vi "Autonomous Independent.vi"() -> ()   [LabVIEW 2017]
doc: "This VI is called when autonomous begins, and will automatically be terminated when autonomous ends. You can carry out timed or sensor driven robot movement independently without needing to return to the caller."
uses:
  <vilib>/Rock Robotics/WPI/RobotDrive/WPI_RobotDriveArcadeDrive_Standard(NoSaturation).vi
  <vilib>/Rock Robotics/Network Tables/NT Read String.vi
  <vilib>/Rock Robotics/Network Tables/NT Write Numeric Array.vi
  <vilib>/Rock Robotics/WPI/ThirdParty/Phoenix-LabVIEW/Motor Controller/Controls/CTRE_Phoenix_MotorControl_FeedbackDevice.ctl
  <vilib>/Rock Robotics/WPI/ThirdParty/Phoenix-LabVIEW/Motor Controller/Controls/CTRE_Phoenix_MotorControl_ControlMode.ctl
panel:
  in  "Output":dbl
  in  "milliseconds to wait":u32
  in  "Acceleration 2":i32
  in  "Cruise Velocity 2":i32
  in  "Invert? Right":bool
  in  "Invert? Left":bool
  in  "Right SensorPhase":bool
  in  "Left SensorPhase":bool
  in  "PIDF":cluster{"P":dbl, "I":dbl, "D":dbl, "F":dbl}
  # "Be sure to right-click and choose Data Operations>>Make Current Value default if you want to save the array values with the VI"
  # "Move 1"
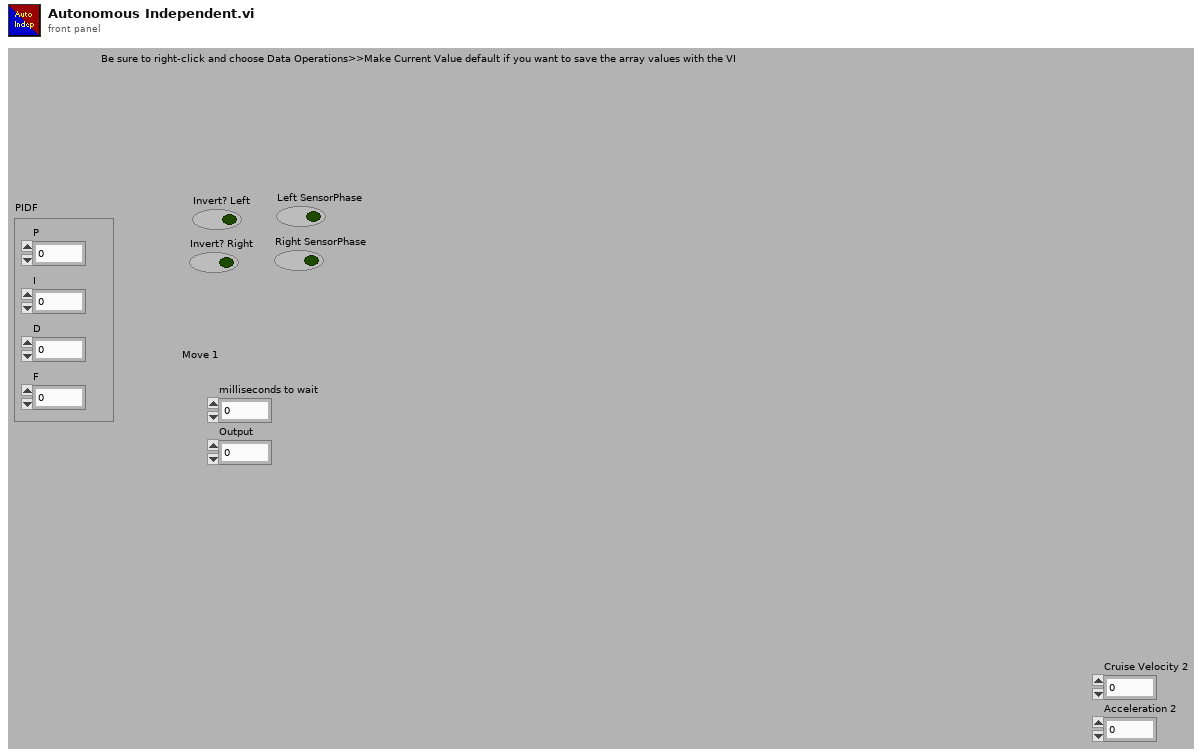
[diagram p1: front panel]
types:
  T1 = typedef "WPI_JoystickDevRef.ctl" = cluster{"Device":T2}
  T2 = typedef "WPI_JoystickDeviceEnum.ctl" = enum16{"USB 0", "USB 1", "USB 2", "USB 3", "USB 4", "USB 5"}
  T3 = typedef "WPI_MotorControlDeviceRef.ctl" = cluster{"DeviceStatus":errorcluster, "Type":T4, "PWM":cluster{"PWM Channel":T5, "DeadBand":T6}, "CAN":cluster{"Device Number":u8, "SetOutput VI Ref":variant, "GetOutput VI Ref":variant, "Enable VI Ref":variant, "Disable VI Ref":variant, "Data":variant}, "Invert":bool, "DIO PWM":cluster{"PWM \"Enable\" Channel":T5, "DIOChannel":T7, "PWM Rate":dbl}}
  T4 = typedef "WPI_MotorControlType.ctl" = enum16{"PWM", "CAN", "DIO PWM"}
  T5 = typedef "FPGA_DIOPWMChannel.ctl" = enum8{"PWM 0", "PWM 1", "PWM 2", "PWM 3", "PWM 4", "PWM 5", "PWM 6", "PWM 7", "PWM 8", "PWM 9", "PWM MXP 0", "PWM MXP 1", "PWM MXP 2", "PWM MXP 3", "PWM MXP 4", "PWM MXP 5", "PWM MXP 6", "PWM MXP 7", "PWM MXP 8", "PWM MXP 9", "Invalid"}
  T6 = typedef "WPI_PWMDeadband.ctl" = cluster{"Name":string, "maxPositivePwm":i32, "minPositivePwm":i32, "centerPwm":i32, "maxNegativePwm":i32, "minNegativePwm":i32, "angularRange":u16}
  T7 = typedef "FPGA_DIOChannel.ctl" = enum8{"DIO 0", "DIO 1", "DIO 2", "DIO 3", "DIO 4", "DIO 5", "DIO 6", "DIO 7", "DIO 8", "DIO 9", "DIO MXP 0", "DIO MXP 1", "DIO MXP 2", "DIO MXP 3", "DIO MXP 4", "DIO MXP 5", "DIO MXP 6", "DIO MXP 7", "DIO MXP 8", "DIO MXP 9", "DIO MXP 10", "DIO MXP 11", "DIO MXP 12", "DIO MXP 13", "DIO MXP 14", "DIO MXP 15", "SPI Port CS1", "SPI Port CS2", "SPI Port CS3", "SPI Port MISO", "SPI Port MOSI", "Invalid"}
  T8 = typedef "CTRE_Phoenix_MotorControl_FeedbackDevice.ctl" = i8
  T9 = typedef "CTRE_Phoenix_MotorControl_ControlMode.ctl" = u16
  T10 = typedef "WPI_RobotDriveDevRef.ctl" = cluster{"DevStatus":errorcluster, "Motors[]":T3[], "Square Inputs":bool, "Max Output":dbl}
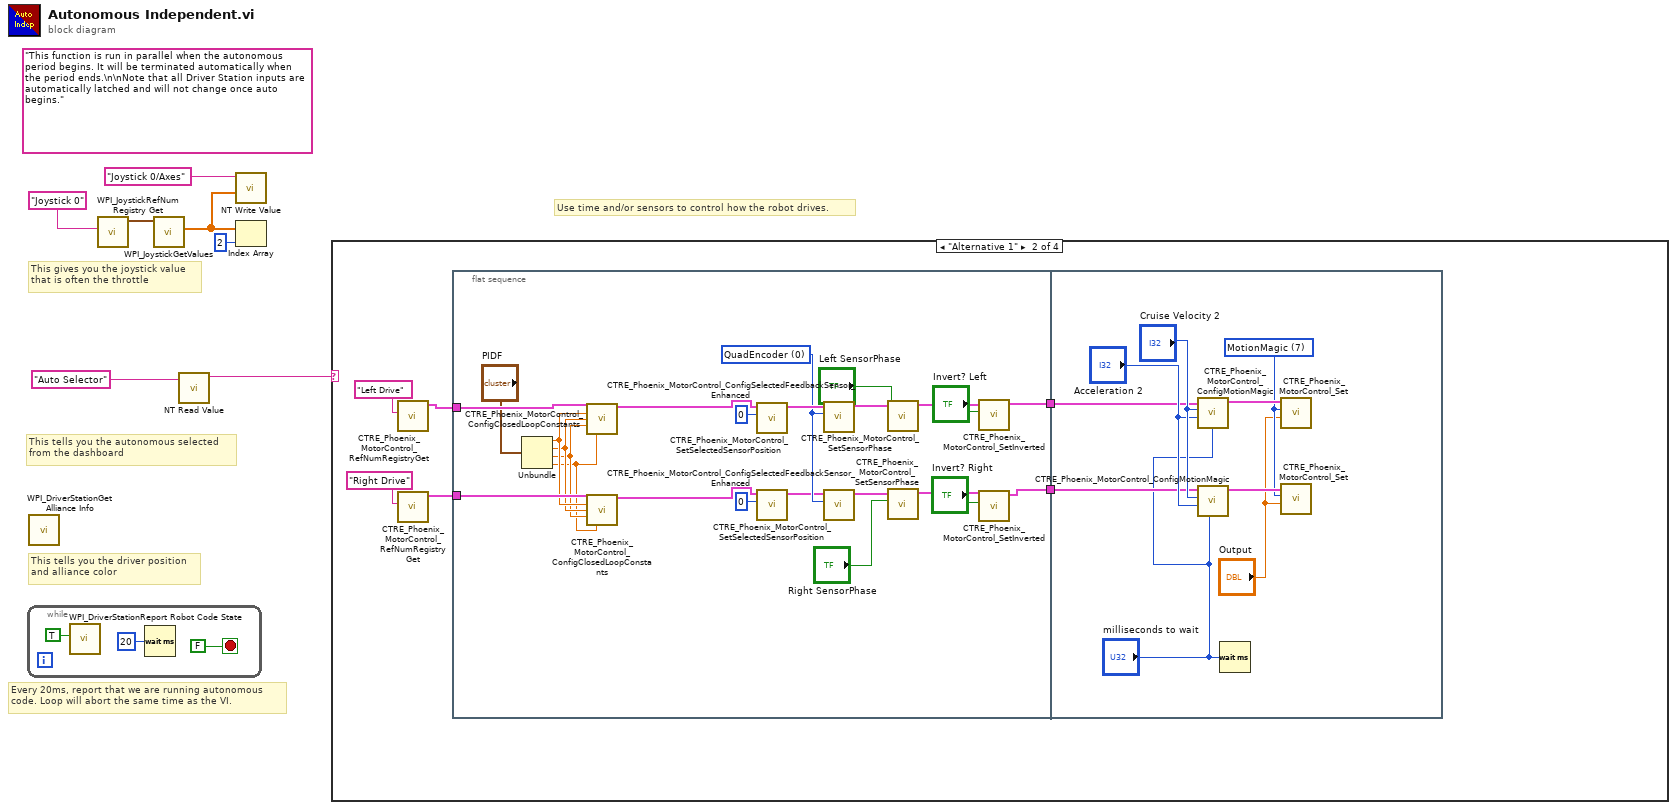
[diagram p0: block diagram]
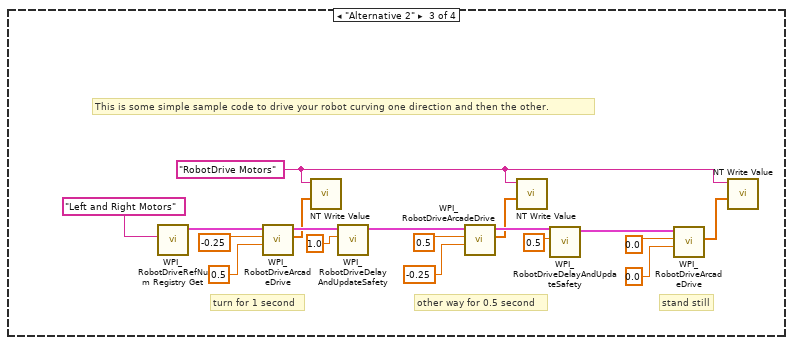
[diagram p3: hidden frame]
diagram:
  (unwired) "This function is run in parallel when the autonomous period begins. It will be terminated automatically when the period ends.\n\nNote that all Driver Station inputs are automatically latched and will not change once auto begins."
  # "This tells you the autonomous selected\nfrom the dashboard"
  # "Every 20ms, report that we are running autonomous\ncode. Loop will abort the same time as the VI."
  # "This gives you the joystick value\nthat is often the throttle"
  # "Use time and/or sensors to control how the robot drives."
  # "This tells you the driver position\nand alliance color"
  n1 = while {
    stop <- FALSE stop-if-true
    n2 = call <vilib>:"WPI_DriverStationReport Robot Code State.vi"("Autonomous"=TRUE) -> ()  [unwired: 10 in, 1 out]
    n3 = Wait (ms)(milliseconds to wait=u32 20) -> ()  [unwired: 1 out]
  }
  n4 = call <vilib>:"WPI_DriverStationGet Alliance Info.vi"() -> ()  [unwired: 12 out]
  n5 = call <vilib>:"WPI_JoystickRefNum Registry Get.vi"("refnum name"="Joystick 0") -> ("JoystickDevRef"=w6:T1)  [unwired: 1 in, 9 out]
  n6 = call <vilib>:"WPI_JoystickGetValues.vi"("JoystickDevRef"=w6) -> ("Axes"=w2:dbl[])  [unwired: 6 in, 4 out]
  n7 = call-poly <vilib>:"NT Read Value.vi"("Name"="Auto Selector") -> ("String"=w3:string)  [unwired: 9 in, 1 out]
  n8 = call-poly <vilib>:"NT Write Value.vi"("Numeric Array"=w2, "Name"="Joystick 0/Axes") -> ()  [unwired: 9 in, 1 out]
  n9 = Index Array(array=w2, index=2) -> ()  [unwired: 1 out]
  n10 = case shown="\"Alternative 1\"" w3 {
    frame Default {
      # "You can put your main auto here, or you can right-click on the case and make any\nother frame be the default case."
      # "This is the frame that will execute if no selection is made, or if it is not recognized"
    }
    frame "Alternative 1" {
      n11 = call <vilib>:"CTRE_Phoenix_MotorControl_RefNumRegistryGet.vi"("refnum name"="Left Drive") -> ("PhoenixMotorControlDevRef"=w14:T3)  [unwired: 9 in, 1 out]
      n12 = call <vilib>:"CTRE_Phoenix_MotorControl_RefNumRegistryGet.vi"("refnum name"="Right Drive") -> ("PhoenixMotorControlDevRef"=w13:T3)  [unwired: 9 in, 1 out]
      n13 = flat-sequence {
        tunnel: w14 -> [w40]
        tunnel: w13 -> [w39]
        tunnel: [w18] -> w12
        tunnel: [w17] -> w11
        tunnel: w12 -> [w47]
        tunnel: w11 -> [w46]
        frame #0 {
          w28 = T8 0 items=["None"=-1, "QuadEncoder"=0, "Analog"=2, "Tachometer"=4, "Pulse Width Encoded Position"=8, "Sensor Sum (S0 + S1)"=9, "Sensor Difference (D0 - D1)"=10, "Remote Source 0"=11, "Remote Source 1"=12, "Software Emulated"=15] ("Feedback Device")
          n14 = Unbundle("PIDF") -> ("P"=w37:dbl, "I"=w36:dbl, "D"=w35:dbl, "F"=w34:dbl)
          n15 = call <vilib>:"CTRE_Phoenix_MotorControl_ConfigClosedLoopConstants.vi"("PhoenixMotorControlDevRef"=w40, "P"=w37, "I"=w36, "D"=w35, "F"=w34) -> ("PhoenixMotorControlDevRef"=w33:T3)  [unwired: 9 in, 1 out]
          n16 = call <vilib>:"CTRE_Phoenix_MotorControl_ConfigClosedLoopConstants.vi"("PhoenixMotorControlDevRef"=w39, "P"=w37, "I"=w36, "D"=w35, "F"=w34) -> ("PhoenixMotorControlDevRef"=w32:T3)  [unwired: 9 in, 1 out]
          n17 = call "CTRE_Phoenix_MotorControl_SetSelectedSensorPosition.vi"("New Sensor Position"=0, "PhoenixMotorControlDevRef"=w33) -> ("PhoenixMotorControlDevRef"=w29:T3)  [unwired: 8 in, 1 out]
          n18 = call "CTRE_Phoenix_MotorControl_SetSelectedSensorPosition.vi"("New Sensor Position"=0, "PhoenixMotorControlDevRef"=w32) -> ("PhoenixMotorControlDevRef"=w27:T3)  [unwired: 8 in, 1 out]
          n19 = call <vilib>:"CTRE_Phoenix_MotorControl_ConfigSelectedFeedbackSensor_Enhanced.vi"("Feedback Device"=w28, "PhoenixMotorControlDevRef"=w29) -> ("PhoenixMotorControlDevRef"=w26:T3)  [unwired: 8 in, 1 out]
          n20 = call <vilib>:"CTRE_Phoenix_MotorControl_ConfigSelectedFeedbackSensor_Enhanced.vi"("Feedback Device"=w28, "PhoenixMotorControlDevRef"=w27) -> ("PhoenixMotorControlDevRef"=w25:T3)  [unwired: 8 in, 1 out]
          n21 = call <vilib>:"CTRE_Phoenix_MotorControl_SetSensorPhase.vi"("PhaseSensor"="Left SensorPhase", "PhoenixMotorControlDevRef"=w26) -> ("PhoenixMotorControlDevRef"=w21:T3)  [unwired: 8 in, 1 out]
          n22 = call <vilib>:"CTRE_Phoenix_MotorControl_SetSensorPhase.vi"("PhaseSensor"="Right SensorPhase", "PhoenixMotorControlDevRef"=w25) -> ("PhoenixMotorControlDevRef"=w22:T3)  [unwired: 8 in, 1 out]
          n23 = call <vilib>:"CTRE_Phoenix_MotorControl_SetInverted.vi"("Invert?"="Invert? Left", "PhoenixMotorControlDevRef"=w21) -> ("PhoenixMotorControlDevRef"=w18:T3)  [unwired: 8 in, 1 out]
          n24 = call <vilib>:"CTRE_Phoenix_MotorControl_SetInverted.vi"("Invert?"="Invert? Right", "PhoenixMotorControlDevRef"=w22) -> ("PhoenixMotorControlDevRef"=w17:T3)  [unwired: 8 in, 1 out]
        }
        frame #1 {
          w42 = T9 7 items=["PercentOutput"=0, "Position"=1, "Velocity"=2, "Current"=3, "Follower"=5, "MotionProfile"=6, "MotionMagic"=7, "MotionMagicArc"=8, "MotionProfileArc"=10, "Disabled"=15] ("Control Mode")
          n25 = call <vilib>:"CTRE_Phoenix_MotorControl_ConfigMotionMagic.vi"("timeoutMs"="milliseconds to wait", "Acceleration"="Acceleration 2", "Cruise Velocity"="Cruise Velocity 2", "PhoenixMotorControlDevRef"=w47) -> ("PhoenixMotorControlDevRef"=w44:T3)  [unwired: 6 in, 1 out]
          n26 = call <vilib>:"CTRE_Phoenix_MotorControl_ConfigMotionMagic.vi"("timeoutMs"="milliseconds to wait", "Acceleration"="Acceleration 2", "Cruise Velocity"="Cruise Velocity 2", "PhoenixMotorControlDevRef"=w46) -> ("PhoenixMotorControlDevRef"=w43:T3)  [unwired: 6 in, 1 out]
          n27 = Wait (ms)(milliseconds to wait="milliseconds to wait") -> ()  [unwired: 1 out]
          n28 = call "CTRE_Phoenix_MotorControl_Set.vi"("Output"="Output", "Control Mode"=w42, "PhoenixMotorControlDevRef"=w44) -> ()  [unwired: 7 in, 2 out]
          n29 = call "CTRE_Phoenix_MotorControl_Set.vi"("Output"="Output", "Control Mode"=w42, "PhoenixMotorControlDevRef"=w43) -> ()  [unwired: 7 in, 2 out]
        }
      }
    }
    frame "Alternative 2" {
      w51 = "RobotDrive Motors" ("Name")
      # "This is some simple sample code to drive your robot curving one direction and then the other."
      # "stand still"
      # "other way for 0.5 second"
      # "turn for 1 second"
      n30 = call <vilib>:"WPI_RobotDriveRefNum Registry Get.vi"("refnum name"="Left and Right Motors") -> ("RobotDriveDevRef"=w67:T10)  [unwired: 1 in, 9 out]
      n31 = call-poly <vilib>:"WPI_RobotDriveArcadeDrive.vi"("Y axis value"=0.5 ("X axis value"), "X axis value"=-0.25, "RobotDriveDevRef"=w67) -> ("Motor Values"=w50:dbl[], "RobotDriveDevRef"=w60:T10)  [unwired: 1 in, 6 out]
      n32 = call-poly <vilib>:"NT Write Value.vi"("Numeric Array"=w50, "Name"=w51) -> ()  [unwired: 9 in, 1 out]
      n33 = call <vilib>:"WPI_RobotDriveDelayAndUpdateSafety.vi"("Delay (s)"=1.0, "RobotDriveDevRef"=w60) -> ("RobotDriveDevRef 2"=w61:T10)  [unwired: 8 in, 1 out]
      n34 = call-poly <vilib>:"WPI_RobotDriveArcadeDrive.vi"("Y axis value"=-0.25 ("X axis value"), "X axis value"=0.5, "RobotDriveDevRef"=w61) -> ("Motor Values"=w52:dbl[], "RobotDriveDevRef"=w62:T10)  [unwired: 1 in, 6 out]
      n35 = call-poly <vilib>:"NT Write Value.vi"("Numeric Array"=w52, "Name"=w51) -> ()  [unwired: 9 in, 1 out]
      n36 = call <vilib>:"WPI_RobotDriveDelayAndUpdateSafety.vi"("Delay (s)"=0.5, "RobotDriveDevRef"=w62) -> ("RobotDriveDevRef 2"=w63:T10)  [unwired: 8 in, 1 out]
      n37 = call-poly <vilib>:"WPI_RobotDriveArcadeDrive.vi"("Y axis value"=0.0 ("X axis value"), "X axis value"=0.0, "RobotDriveDevRef"=w63) -> ("Motor Values"=w53:dbl[])  [unwired: 1 in, 7 out]
      n38 = call-poly <vilib>:"NT Write Value.vi"("Numeric Array"=w53, "Name"=w51) -> ()  [unwired: 9 in, 1 out]
    }
    frame "Your Turn" {
    }
  }
